vi "Read Data IDs.vi"(8 "error in (no error)":errorcluster, 11 "Single_Array in":refnum<class "Single_Array.lvclass">) -> (0 "error out":errorcluster, 2 "Data IDs":string[](array[string]), 3 "Single_Array out":refnum<class "Single_Array.lvclass">)   [LabVIEW 2016, in "Base Data Class.lvlib" / "Single_Array.lvclass"]
uses:
  Single_Array.lvclass
  Single_Array.lvclass/Single_Array.ctl
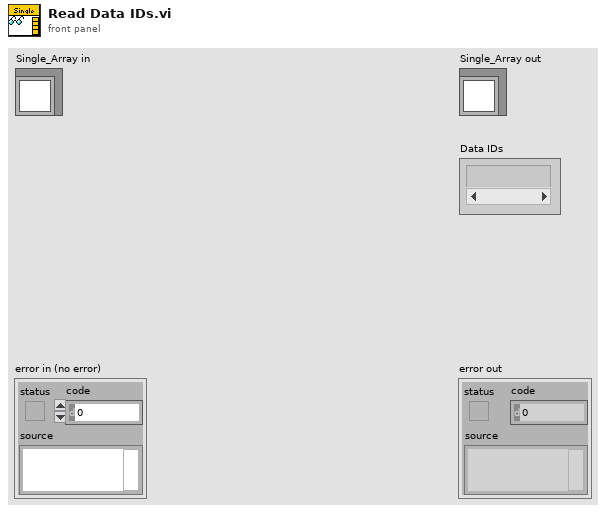
[diagram p1: front panel]
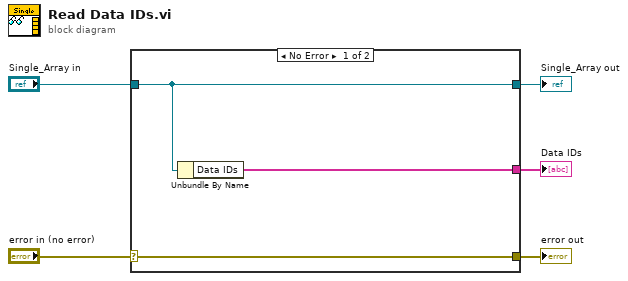
[diagram p0: block diagram]
diagram:
  n1 = case shown="No Error" "error in (no error)" {
    selector: "error in (no error)" -> [w8 w9]
    tunnel: [w8 w9] -> w4
    tunnel: [w7 w10] -> w2
    tunnel: "Single_Array in" -> [w7 w10]
    tunnel: [w6 _] -> w1
    frame No Error {
      n2 = Unbundle By Name(w7) -> ("Data IDs"=w6:string[])
    }
    frame Error {
    }
  }
  "error out" <- w4
  "Single_Array out" <- w2
  "Data IDs" <- w1
